vi "solar_excel Worksheet Range.vi"(8 "error in (no error)":errorcluster, 11 "Excel Worksheet in":T1) -> (0 "error out":errorcluster, 1 "Columns":u32, 2 "Rows":u32, 3 "Excel Worksheet out":T1)   [LabVIEW 2018]
doc: "This returns the row and column range count. Note: The range count may be larger than the content, use the Truncate Cells VI to remove empty cells at the end."
uses:
  solar_excel_ctl Worksheet.ctl
  solar_excel_ctl TSV.ctl
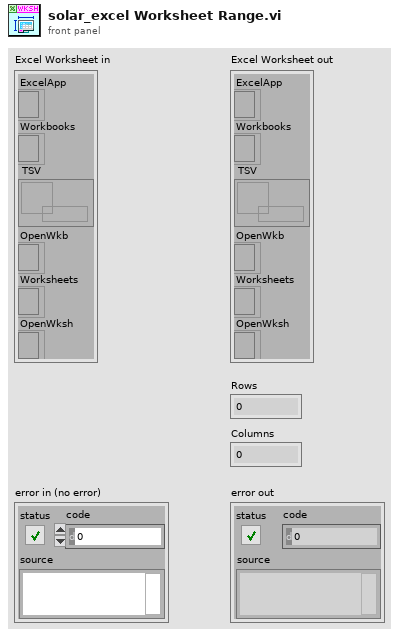
[diagram p1: front panel]
types:
  T1 = typedef "solar_excel_ctl Worksheet.ctl" = cluster{"ExcelApp":refnum<k7>, "Workbooks":refnum<k7>, "TSV":refnum<queue>, "OpenWkb":refnum<k7>, "Worksheets":refnum<k7>, "OpenWksh":refnum<k7>}
  T2 = typedef "solar_excel_ctl TSV.ctl" = cluster{"Path":path, "Dirty":bool, "ActiveSheet":u8, "Worksheets":string[], "Worksheet Cells":cluster{"Cells":string[][]}[]}
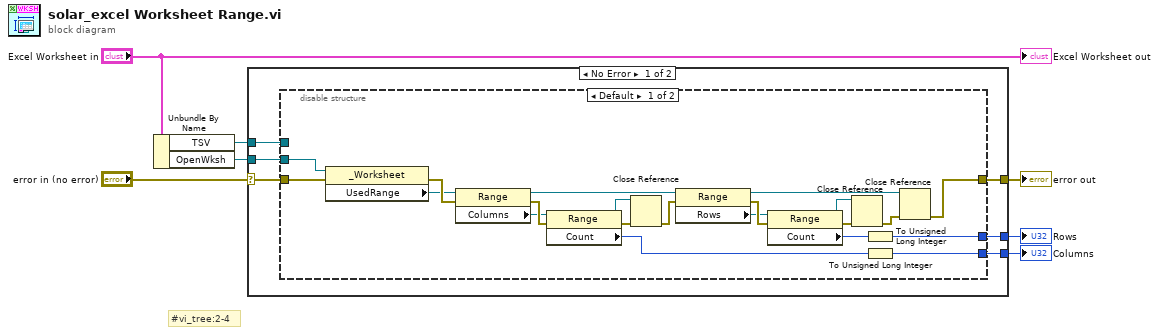
[diagram p0: block diagram]
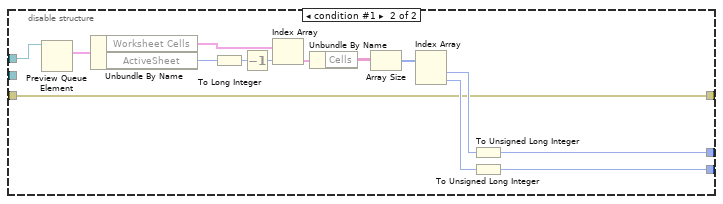
[diagram p2: hidden frame]
diagram:
  # "#vi_tree:2-4"
  n1 = Unbundle By Name("Excel Worksheet in") -> ("TSV"=w1:refnum<queue>, "OpenWksh"=w5:refnum<k7>)
  n2 = case shown="No Error" "error in (no error)" {
    selector: "error in (no error)" -> [w13 w49]
    tunnel: [w11 w49] -> w7
    tunnel: w5 -> [w12 _]
    tunnel: [w10 _] -> w3
    tunnel: [w9 _] -> w2
    tunnel: w1 -> [w8 _]
    frame No Error {
      n3 = disable-structure shown="Default" {
        disable-tunnel: w13 -> [w34 w35]
        disable-tunnel: w12 -> [w33 _]
        disable-tunnel: [w19 w35] -> w11
        disable-tunnel: [w15 w38] -> w10
        disable-tunnel: [w14 w36] -> w9
        disable-tunnel: w8 -> [_ w44]
        frame condition #0 (active) {
          n4 = property class="_Worksheet"(reference=w33, error in=w34) -> (error out=w32:errorcluster, "UsedRange"=w31:refnum<k7>)  [unwired: 1 out]
          n5 = property class="Range"(reference=w31, error in=w32) -> (reference out=w22:refnum<k7>, error out=w30:errorcluster, "Columns"=w29:refnum<k7>)
          n6 = property class="Range"(reference=w29, error in=w30) -> (reference out=w27:refnum<k7>, error out=w28:errorcluster, "Count"=w16:i32)
          n7 = Close Reference(reference=w27, error in (no error)=w28) -> (error out=w24:errorcluster)
          n8 = property class="Range"(reference=w22, error in=w24) -> (reference out=w18:refnum<k7>, error out=w23:errorcluster, "Rows"=w21:refnum<k7>)
          n9 = property class="Range"(reference=w21, error in=w23) -> (reference out=w26:refnum<k7>, error out=w25:errorcluster, "Count"=w17:i32)
          n10 = Close Reference(reference=w26, error in (no error)=w25) -> (error out=w20:errorcluster)
          n11 = To Unsigned Long Integer(number=w17) -> (unsigned 32bit integer=w15:u32)
          n12 = To Unsigned Long Integer(number=w16) -> (unsigned 32bit integer=w14:u32)
          n13 = Close Reference(reference=w18, error in (no error)=w20) -> (error out=w19:errorcluster)
        }
        frame condition #1 {
          n14 = Preview Queue Element(queue=w44) -> (element=w43:T2)  [unwired: 2 in, 3 out]
          n15 = Unbundle By Name(w43) -> ("Worksheet Cells"=w48:cluster{"Cells":string[][]}[], "ActiveSheet"=w47:u8)
          n16 = To Long Integer(number=w47) -> (32bit integer=w45:i32)
          n17 = Decrement(x=w45) -> (x-1=w46:i32)
          n18 = Index Array(array=w48, index=w46) -> (element=w42:cluster{"Cells":string[][]})
          n19 = Unbundle By Name(w42) -> ("Cells"=w41:string[][])
          n20 = Array Size(array=w41) -> (size(s)=w40:i32[])
          n21 = Index Array(array=w40) -> (element #1=w39:i32, element #2=w37:i32)  [unwired: 2 in]
          n22 = To Unsigned Long Integer(number=w39) -> (unsigned 32bit integer=w38:u32)
          n23 = To Unsigned Long Integer(number=w37) -> (unsigned 32bit integer=w36:u32)
        }
      }
    }
    frame Error {
    }
  }
  "error out" <- w7
  "Rows" <- w3
  "Columns" <- w2
  "Excel Worksheet out" <- "Excel Worksheet in"
